vi "CalculateUncertainties.vi"(8 "error in (no error)":errorcluster, 9 "Normalized number of Droplets vs. Temperature All Data":cluster{dbl[], dbl[]}(graph), 11 "Array of Different Experiments":cluster{T1}[](array[cluster])) -> (0 "error out":errorcluster, 3 "Uncertainties":dbl[](array[numeric]))   [LabVIEW 2015]
doc: "Use this template to build a VI to use as a subVI."
uses:
  TypeDef/MultipleFileData.ctl
  <vilib>/Analysis/NI_AALBase.lvlib
panel:
  out "Array 4":i32[][](array[numeric])
  out "Array 3":dbl[][](array[numeric])
  out "Array 2":dbl[](array[numeric])
  out "Array":dbl[][](array[numeric])
  out "Numeric":i32
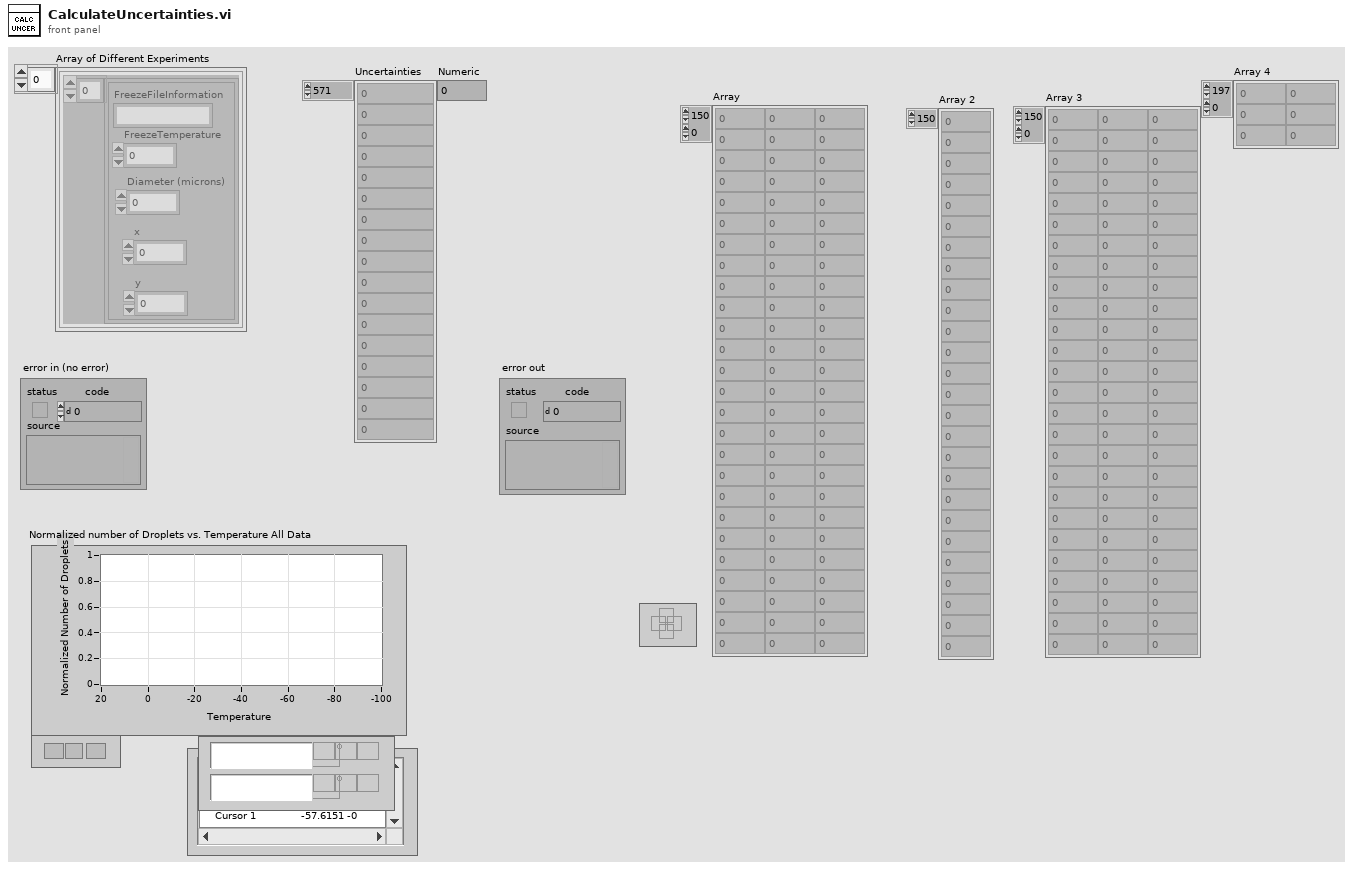
[diagram p1: front panel]
types:
  T1 = typedef "MultipleFileData.ctl" = cluster{"FreezeTemperature":dbl, "FreezeFileInformation":string, "Diameter (microns)":dbl, "x":sgl, "y":sgl}[]
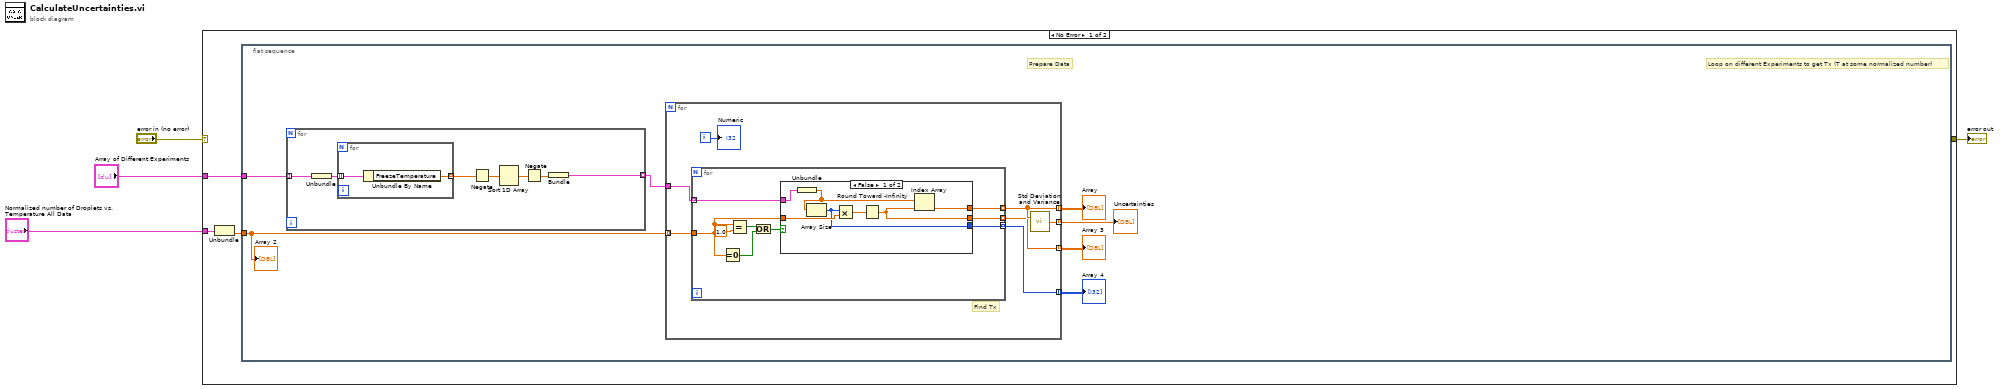
[diagram p0: block diagram]
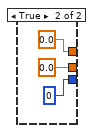
[diagram p2: hidden frame]
diagram:
  n1 = case shown="No Error" "error in (no error)" {
    selector: "error in (no error)" -> [_ w50]
    tunnel: [_ w50] -> w3
    tunnel: "Array of Different Experiments" -> [w7 _]
    tunnel: "Normalized number of Droplets vs. Temperature All Data" -> [w6 _]
    frame No Error {
      n2 = Unbundle(w6) -> (w5:dbl[])  [unwired: 1 out]
      n3 = flat-sequence {
        tunnel: w7 -> [w9]
        tunnel: w5 -> [w14]
        frame #0 {
          # "Prepare Data"
          # "Loop on different Experiments to get Tx (T at some normalized number)"
          n4 = for {
            tunnel: w9 -> [w21] mode=indexing
            tunnel: [w15] -> w8 mode=indexing
            n5 = Unbundle(w21) -> (w20:T1)
            n6 = for {
              tunnel: w20 -> [w23] mode=indexing
              tunnel: [w22] -> w17 mode=indexing
              n7 = Unbundle By Name(w23) -> ("FreezeTemperature"=w22:dbl)
            }
            n8 = Negate(x=w17) -> (-x=w19:dbl[])
            n9 = Sort 1D Array(array=w19) -> (sorted array=w18:dbl[])
            n10 = Negate(x=w18) -> (-x=w16:dbl[])
            n11 = Bundle(w16) -> (w15:cluster{dbl[]})  [unwired: 1 in]
          }
          n12 = for {
            tunnel: w8 -> [w30]
            tunnel: w14 -> [w29] mode=indexing
            tunnel: [w28] -> w13 mode=indexing
            tunnel: [w26] -> w12 mode=indexing
            tunnel: [w25] -> w11 mode=indexing
            tunnel: [w24] -> w10 mode=indexing
            i -> [w27]
            # "Find Tx"
            n13 = for {
              tunnel: w30 -> [w39] mode=indexing
              tunnel: w29 -> [w36]
              tunnel: [w38] -> w26 mode=indexing
              tunnel: [w32] -> w25 mode=indexing
              tunnel: [w31] -> w24 mode=indexing
              n14 = Equal To 0?(x=w36) -> (x = 0?=w34:bool)
              n15 = Equal?(x=w36, y=1.0) -> (x = y?=w35:bool)
              n16 = Or(x=w35, y=w34) -> (x .or. y?=w33:bool)
              n17 = case shown="False" w33 {
                tunnel: w39 -> [w42 _]
                tunnel: w36 -> [w46 _]
                tunnel: [w43 0.0 ("FreezeTemperature")] -> w38
                tunnel: [w40 0.0] -> w32
                tunnel: [w44 0] -> w31
                frame False {
                  n18 = Unbundle(w42) -> (w41:dbl[])
                  n19 = Array Size(array=w41) -> (size(s)=w44:i32)
                  n20 = Multiply(x=w44, y=w46) -> (x*y=w45:dbl)
                  n21 = Round Toward -Infinity(1:w45) -> (0:w40:dbl)
                  n22 = Index Array(array=w41, index=w40) -> (element=w43:dbl)
                }
                frame True {
                }
              }
            }
            n23 = call <vilib>:"Std Deviation and Variance.vi"("X"=w26) -> ("standard deviation"=w28:dbl)  [unwired: 1 in, 2 out]
            "Numeric" <- w27
          }
          "Uncertainties" <- w13
          "Array" <- w12
          "Array 3" <- w11
          "Array 4" <- w10
          "Array 2" <- w14
        }
      }
    }
    frame Error {
    }
  }
  "error out" <- w3
